vi "sio write.vi"(9 "len":i32, 10 "buf":string, 11 "port":i32) -> (1 "buf out":string, 2 "Status":i32, 3 "port out":i32)   [LabVIEW 2015, in "PCOMM.lvlib"]
doc: "int WINAPI sio_write(int port, char *buf, int len);"
uses:
  PCOMM.lvlib
  PCOMM.DLL
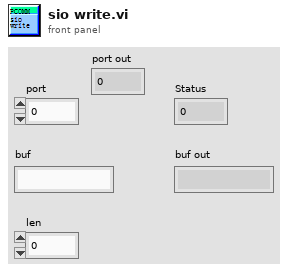
[diagram p1: front panel]
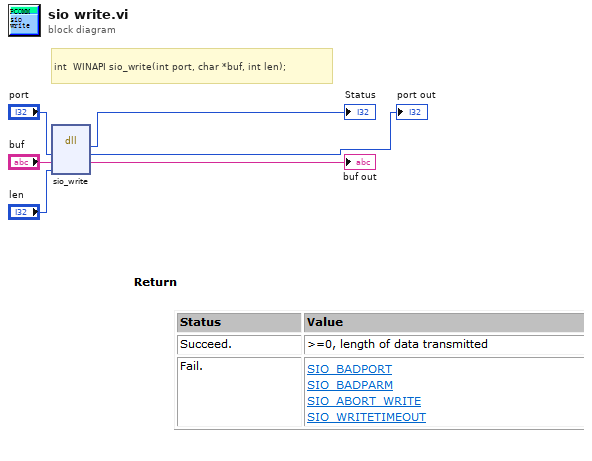
[diagram p0: block diagram]
diagram:
  # "int  WINAPI sio_write(int port, char *buf, int len);"
  n1 = dll-call lib="PTH2Yabs EDesktopLabview串口助手串口助手2.0Ing10_v3.2.0libpcommPCOMM.*" fn="sio_write"("port"="port", "buf"="buf", "len"="len") -> (→"Status":i32, "port"=→"port out":i32, "buf"=→"buf out":string)  [unwired: 4 in, 2 out]
